vi "Example2-Globals.vi"() -> ()   [LabVIEW 2020]
doc: "Example of use global and shared variable."
uses:
  Ctrls/DataCluster.ctl
  Ctrls/GlobalStop.vi
panel:
  in  "Calculate":bool
  in  "C":i8(knob) scale=0.0..10.0
  in  "B":i8(knob) scale=0.0..10.0
  in  "A":i8(knob) scale=0.0..10.0
  in  "stop":bool
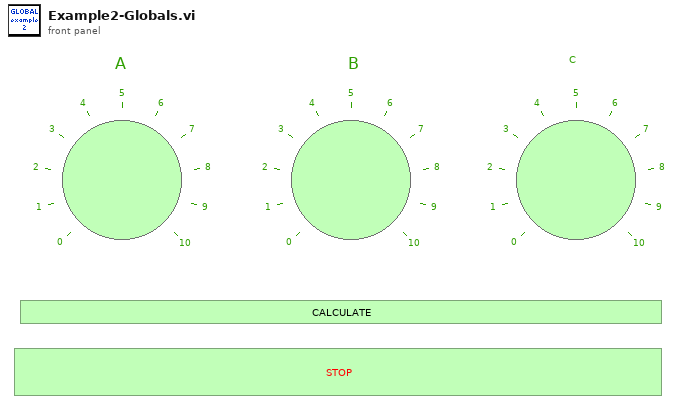
[diagram p1: front panel]
types:
  T1 = typedef "DataCluster.ctl" = cluster{"DataAndTime":timestamp, "Log message ":string, "Parameter 1":dbl}
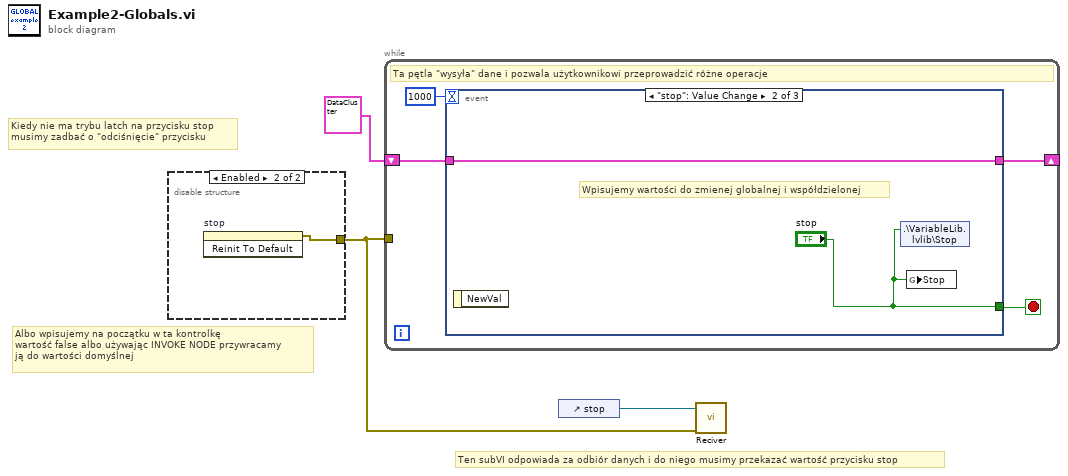
[diagram p0: block diagram]
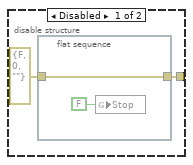
[diagram p2: hidden frame]
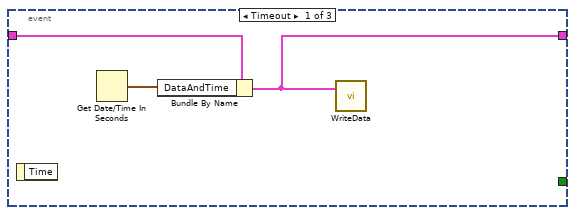
[diagram p3: hidden frame]
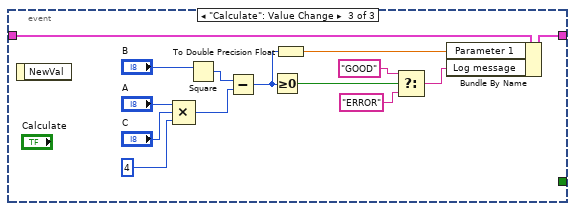
[diagram p4: hidden frame]
diagram:
  # "Albo wpisujemy na początku w ta kontrolkę \nwartość false albo używając INVOKE NODE przywracamy\nją do wartości domyślnej"
  # "Kiedy nie ma trybu latch na przycisku stop \nmusimy zadbać o \"odciśnięcie\" przycisku"
  # "Ten subVI odpowiada za odbiór danych i do niego musimy przekazać wartość przycisku stop"
  n1 = disable-structure shown="Enabled" {
    disable-tunnel: [w5 w8] -> w1
    frame Disabled {
      n2 = flat-sequence {
        tunnel: errorcluster {"status"=FALSE, "code"=0, "source"=""} ("error out") -> [w7]
        tunnel: [w7] -> w5
        frame #0 {
          n3 = global write "GlobalStop.vi" "Stop"(FALSE ("Stop")) -> ()
        }
      }
    }
    frame Enabled {
      n4 = invoke on="stop" class="Bool (strict)" method="Reinit To Default"() -> (error out=w8:errorcluster)  [unwired: 3 in, 2 out]
    }
  }
  n5 = while {
    shift-right: [w10] -> _
    shift-left: T1 {"DataAndTime"=timestamp(0 s since 1904-01-01), "Log message "="OK", "Parameter 1"=100.0} ("Data In") -> [w9]
    tunnel: w1 -> [_]
    stop <- w11 stop-if-true
    # "Ta pętla \"wysyła\" dane i pozwala użytkownikowi przeprowadzić różne operacje"
    n6 = event shown="[1] \"stop\": Value Change" {
      selector: _ -> [_ _ _]
      dyn-events: _ -> [_ _ _]
      timeout: 1000 ("Numeric") -> [_ _ _]
      tunnel: [_ "stop" _] -> w11
      tunnel: [w13 w17 w24] -> w10
      tunnel: w9 -> [w14 w17 w25]
      event Timeout {
        n7 = event-data() -> ()  [unwired: 1 in, 1 out]
        n8 = Get Date/Time In Seconds() -> (seconds since 1Jan1904=w15:timestamp)
        n9 = Bundle By Name(cluster=w14, "DataAndTime"=w15) -> (w13:T1)
        n10 = call "WriteData.vi"("Data In"=w13) -> ()  [unwired: 3 in]
      }
      event "stop": Value Change {
        # "Wpisujemy wartości do zmienej globalnej i współdzielonej"
        n11 = event-data() -> ()  [unwired: 1 in, 1 out]
        n12 = shared-variable ".\\VariableLib.lvlib\\Stop"("stop") -> ()  [unwired: 1 in, 1 out]
        n13 = global write "GlobalStop.vi" "Stop"("stop") -> ()
      }
      event "Calculate": Value Change {
        n14 = event-data() -> ()  [unwired: 1 in, 1 out]
        n15 = Compound Arithmetic op=MULTIPLY("A", "C", i8 4 ("value")) -> (w27:i8)
        n16 = Square(x="B") -> (x^2=w30:i8)
        n17 = Subtract(x=w30, y=w27) -> (x-y=w19:i8)
        n18 = Greater Or Equal To 0?(x=w19) -> (x >= 0?=w20:bool)
        n19 = To Double Precision Float(number=w19) -> (double precision float=w18:dbl)
        n20 = Select(t="GOOD", s=w20, f="ERROR") -> (s? t:f=w21:string)
        n21 = Bundle By Name(cluster=w25, "Parameter 1"=w18, "Log message"=w21) -> (w24:T1)
      }
    }
  }
  n22 = control-ref of="stop"() -> (w2:refnum<vi>)
  n23 = call "Reciver.vi"("Error In"=w1, "Ref boolean in"=w2) -> ()  [unwired: 9 in, 1 out]
